vi "Motor PWM.vi"(10 "M?":i16, 11 "Pwm":dbl) -> ()   [LabVIEW 2019]
uses:
  <vilib>/myRIO/Instrument Drivers/Onboard IO/PWM/typedefs/PWM Reference.ctl
  <vilib>/myRIO/Common/Instrument Driver Framework/Utilities/typedefs/myRIO Generic Hardware Reference.ctl
  <vilib>/myRIO/Common/Instrument Driver Framework/Utilities/typedefs/Hardware Version Enum.ctl
  <vilib>/myRIO/Common/Instrument Driver Framework/Utilities/typedefs/myRIO v1.0 Reference.ctl
  <vilib>/myRIO/Common/Instrument Driver Framework/Utilities/typedefs/Generic FPGA Reference.ctl
  <vilib>/myRIO/Common/Instrument Driver Framework/myRIO v1.0/PWM/typedefs/PWM Channels Enum.ctl
  <vilib>/myRIO/Instrument Drivers/Onboard IO/PWM/typedefs/PWM Configuration.ctl
  <vilib>/userDefined/High Color/nirio_resource_hc.ctl
  <vilib>/myRIO/Common/Instrument Driver Framework/Utilities/vis/Is FPGA Ref Available.vi
  <vilib>/myRIO/Common/Instrument Driver Framework/myRIO v1.0/PWM/vis/myRIO v1.1 Open PWM.vi
  <vilib>/myRIO/Instrument Drivers/Onboard IO/PWM/vis/Set Duty Cycle and Frequency.vi
  <vilib>/myRIO/Common/Instrument Driver Framework/Utilities/vis/Validate Channels.vi
  <vilib>/myRIO/Common/Instrument Driver Framework/myRIO v1.0/PWM/vis/myRIO v1.0 Reserve PWM.vi
  <vilib>/myRIO/Common/Instrument Driver Framework/myRIO v1.0/PWM/vis/myRIO v1.0 Build MUX Configuration PWM.vi
  <vilib>/myRIO/Common/Instrument Driver Framework/myRIO v1.0/Resource Manager/vis/myRIO v1.0 Reserve Channel List.vi
  <vilib>/myRIO/Common/Instrument Driver Framework/myRIO v1.0/Resource Manager/vis/myRIO v1.0 Create Configuration List.vi
  <vilib>/myRIO/Common/Instrument Driver Framework/myRIO v1.0/Resource Manager/vis/myRIO v1.0 Reserve Channel.vi
  <vilib>/myRIO/Common/Instrument Driver Framework/myRIO v1.0/Resource Manager/vis/myRIO v1.0 Unreserve Channel.vi
  <vilib>/myRIO/Common/Instrument Driver Framework/myRIO v1.0/Resource Manager/vis/myRIO v1.0 Build Mutex Name.vi
  <vilib>/Utility/VariantDataType/GetNumericInfo.vi
  <vilib>/Utility/error.llb/Error Cluster From Error Code.vi
  <vilib>/myRIO/Common/Instrument Driver Framework/myRIO v1.0/myRIO v1.1 Open.vi
  <vilib>/myRIO/Common/Instrument Driver Framework/Utilities/vis/IO Manager.vi
  <vilib>/myRIO/Common/Instrument Driver Framework/Utilities/vis/Configuration Manager.vi
  <vilib>/myRIO/Common/Instrument Driver Framework/myRIO v1.0/Resource Manager/vis/myRIO v1.0 Configure IO.vi
  <vilib>/myRIO/Common/Instrument Driver Framework/myRIO v1.0/myRIO v1.0 Close.vi
  <vilib>/myRIO/Common/Instrument Driver Framework/myRIO v1.0/PWM/vis/myRIO v1.0 Write PWM.vi
  <vilib>/myRIO/Express VI/Onboard IO/PWM/PWM Express VI.xnode
  <vilib>/myRIO/Instrument Drivers/Onboard IO/PWM/vis/myRIO PWM Open.xnode
  <vilib>/myRIO/Instrument Drivers/Onboard IO/PWM/PWM.lvlib
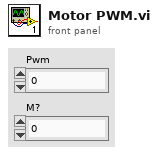
[diagram p1: front panel]
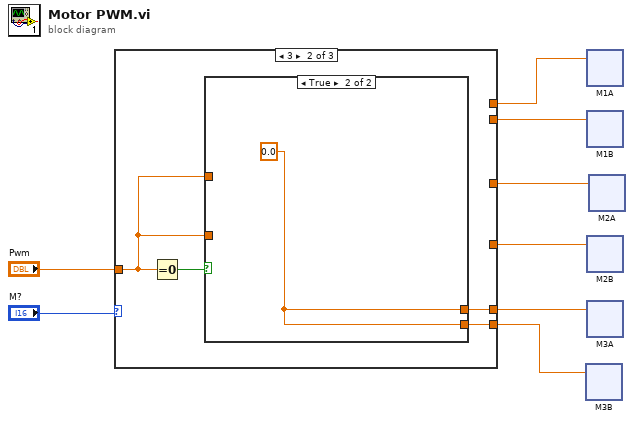
[diagram p0: block diagram]
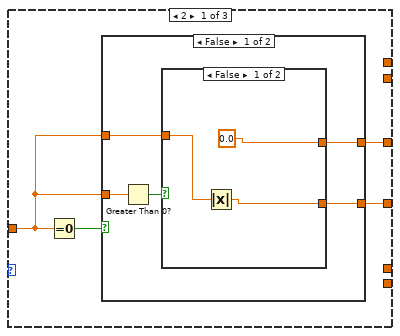
[diagram p2: hidden frame]
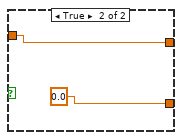
[diagram p3: hidden frame]
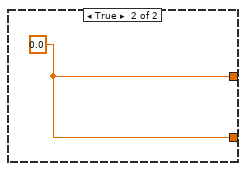
[diagram p4: hidden frame]
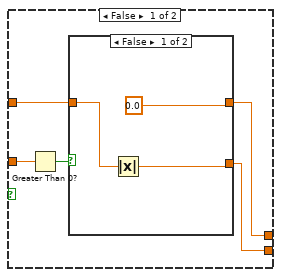
[diagram p5: hidden frame]
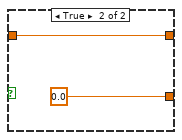
[diagram p6: hidden frame]
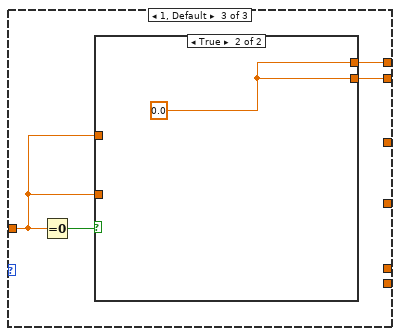
[diagram p7: hidden frame]
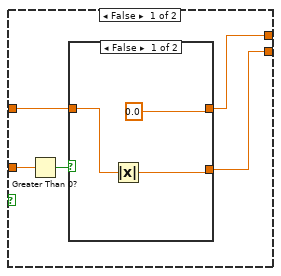
[diagram p8: hidden frame]
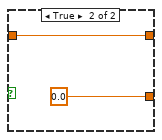
[diagram p9: hidden frame]
diagram:
  n1 = case shown="3" "M?" {
    tunnel: "Pwm" -> [w11 w26 w41]
    tunnel: [_ _ w40] -> w6
    tunnel: [_ _ w39] -> w5
    tunnel: [w10 _ _] -> w4
    tunnel: [w9 _ _] -> w3
    tunnel: [_ w25 _] -> w2
    tunnel: [_ w24 _] -> w1
    frame 2 {
      n2 = Equal To 0?(x=w11) -> (x = 0?=w12:bool)
      n3 = case shown="False" w12 {
        tunnel: w11 -> [w17 _]
        tunnel: w11 -> [w15 _]
        tunnel: [w14 w23] -> w10
        tunnel: [w13 w23] -> w9
        frame False {
          n4 = Greater Than 0?(x=w17) -> (x > 0?=w16:bool)
          n5 = case shown="False" w16 {
            tunnel: w15 -> [w20 w21]
            tunnel: [0.0 ("Duty Cycle") w21] -> w14
            tunnel: [w18 0.0 ("Duty Cycle")] -> w13
            frame False {
              n6 = Absolute Value(x=w20) -> (abs(x)=w18:dbl)
            }
            frame True {
            }
          }
        }
        frame True {
          w23 = 0.0 ("Duty Cycle")
        }
      }
    }
    frame 3 {
      n7 = Equal To 0?(x=w26) -> (x = 0?=w27:bool)
      n8 = case shown="True" w27 {
        tunnel: w26 -> [w32 _]
        tunnel: w26 -> [w30 _]
        tunnel: [w28 w38] -> w25
        tunnel: [w29 w38] -> w24
        frame False {
          n9 = Greater Than 0?(x=w32) -> (x > 0?=w31:bool)
          n10 = case shown="False" w31 {
            tunnel: w30 -> [w35 w36]
            tunnel: [w33 0.0 ("Duty Cycle")] -> w29
            tunnel: [0.0 ("Duty Cycle") w36] -> w28
            frame False {
              n11 = Absolute Value(x=w35) -> (abs(x)=w33:dbl)
            }
            frame True {
            }
          }
        }
        frame True {
          w38 = 0.0 ("Duty Cycle")
        }
      }
    }
    frame 1, Default {
      n12 = Equal To 0?(x=w41) -> (x = 0?=w42:bool)
      n13 = case shown="True" w42 {
        tunnel: w41 -> [w47 _]
        tunnel: w41 -> [w45 _]
        tunnel: [w44 w53] -> w40
        tunnel: [w43 w53] -> w39
        frame False {
          n14 = Greater Than 0?(x=w47) -> (x > 0?=w46:bool)
          n15 = case shown="False" w46 {
            tunnel: w45 -> [w50 w52]
            tunnel: [0.0 ("Duty Cycle") w52] -> w44
            tunnel: [w48 0.0 ("Duty Cycle")] -> w43
            frame False {
              n16 = Absolute Value(x=w50) -> (abs(x)=w48:dbl)
            }
            frame True {
            }
          }
        }
        frame True {
          w53 = 0.0 ("Duty Cycle")
        }
      }
    }
  }
  n17 = xnode "M3B"("Duty Cycle"=w1) -> ()  [unwired: 1 in, 1 out]
  n18 = xnode "M1A"("Duty Cycle"=w6) -> ()  [unwired: 1 in, 1 out]
  n19 = xnode "M1B"("Duty Cycle"=w5) -> ()  [unwired: 1 in, 1 out]
  n20 = xnode "M2B"("Duty Cycle"=w3) -> ()  [unwired: 1 in, 1 out]
  n21 = xnode "M3A"("Duty Cycle"=w2) -> ()  [unwired: 1 in, 1 out]
  n22 = xnode "M2A"("Duty Cycle"=w4) -> ()  [unwired: 1 in, 1 out]
